vi "GP_PSD9.vi"(0 "ConexPSD Reference":refnum<k24>, 1 "error out":errorcluster, 2 "Component ID":i32, 3 "Adress":dbl=1.0, 5 "shot average":dbl=1.0) -> (13 "errstring 2":string, 14 "ConexPSD Reference 2":refnum<k24>, 15 "error out 2":errorcluster caption="error out", 16 "Component ID 2":i32, 17 "PositionX":dbl=1.097, 18 "PositionY":dbl=0.9222, 19 "LaserPower":dbl=1.562)   [LabVIEW 2010]
uses:
  C:/Users/NBTP/Desktop/Tai Anh/Tools Project/LabVIEW/노트북LabVIEW/THz Time/THz Time(SR830_VC_CONEXAGP_nPt_Shot202_2Pt__LGS/Dll/Newport.CONEXPSD.CommandInterface.DLL
  노트북LabVIEW/THz Time/THz Time(SR830_VC_CONEXAGP_nPt_Shot202_2Pt__LGS/Dll/Newport.CONEXPSD.CommandInterface.DLL
panel:
  in  "긴급 정지":bool
  # "Input"
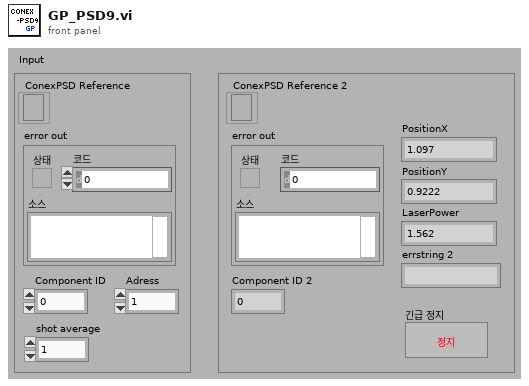
[diagram p1: front panel]
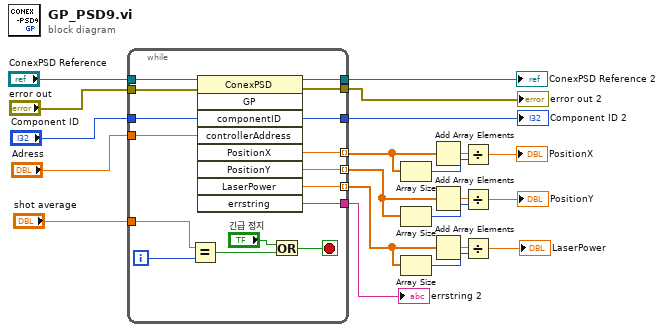
[diagram p0: block diagram]
diagram:
  n1 = while {
    tunnel: "ConexPSD Reference" -> [w36]
    tunnel: [w35] -> w3
    tunnel: [w34] -> w2
    tunnel: "Component ID" -> [w22]
    tunnel: "error out" -> [w33]
    tunnel: "Adress" -> [w32]
    tunnel: [w31] -> w14 mode=indexing
    tunnel: [w30] -> w9 mode=indexing
    tunnel: [w29] -> w8 mode=indexing
    tunnel: "shot average" -> [w28]
    tunnel: [w23] -> w4
    tunnel: [w22] -> w1
    i -> [w27]
    stop <- w24 stop-if-true
    n2 = Equal?(x=w28, y=w27) -> (x = y?=w26:bool)
    n3 = invoke class="ConexPSD" method="GP"(reference=w36, error in=w33, "componentID"=w22, "controllerAddress"=w32) -> (reference out=w35:refnum<k24>, error out=w34:errorcluster, "PositionX"=w31:dbl, "PositionY"=w30:dbl, "LaserPower"=w29:dbl, "errstring"=w23:string)  [unwired: 5 in, 3 out]
    n4 = Or(x="긴급 정지", y=w26) -> (x .or. y?=w24:bool)
  }
  "errstring 2" <- w4
  "ConexPSD Reference 2" <- w3
  "error out 2" <- w2
  "Component ID 2" <- w1
  n5 = Array Size(array=w14) -> (size(s)=w17:i32)
  n6 = Array Size(array=w9) -> (size(s)=w12:i32)
  n7 = Array Size(array=w8) -> (size(s)=w11:i32)
  n8 = Add Array Elements(numeric array=w14) -> (sum=w16:dbl)
  n9 = Add Array Elements(numeric array=w9) -> (sum=w13:dbl)
  n10 = Add Array Elements(numeric array=w8) -> (sum=w10:dbl)
  n11 = Divide(x=w16, y=w17) -> (x/y=→"PositionX":dbl)
  n12 = Divide(x=w13, y=w12) -> (x/y=→"PositionY":dbl)
  n13 = Divide(x=w10, y=w11) -> (x/y=→"LaserPower":dbl)
